vi "16bitImageglobal.vi"(4 "Enum":T3(ring), 5 "Palette Number (gray)":T1(ring), 7 "plane":u32, 8 "router":u8) -> (0 "Palette Number (gray) 2":T1(ring), 1 "Title":string, 2 "error out":errorcluster, 3 "Image Out (duplicate)":T2)   [LabVIEW 2009]
uses:
  <vilib>/vision/Image Controls.llb/IMAQ Image.ctl
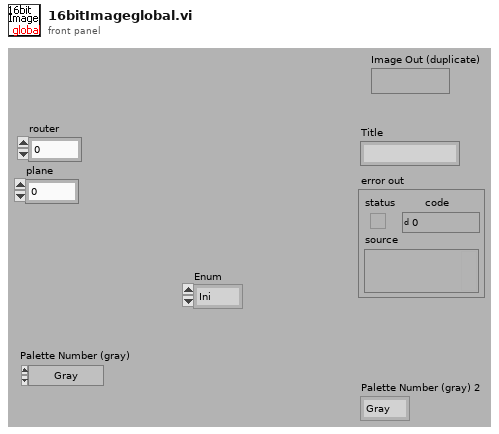
[diagram p1: front panel]
types:
  T1 = enum32{"Gray", "Binary", "Gradient", "Rainbow", "Temperature"}
  T2 = typedef "IMAQ Image.ctl" = refnum<image>
  T3 = enum16{"Ini", "Dump", "Colorpal", "Input", "Get"}
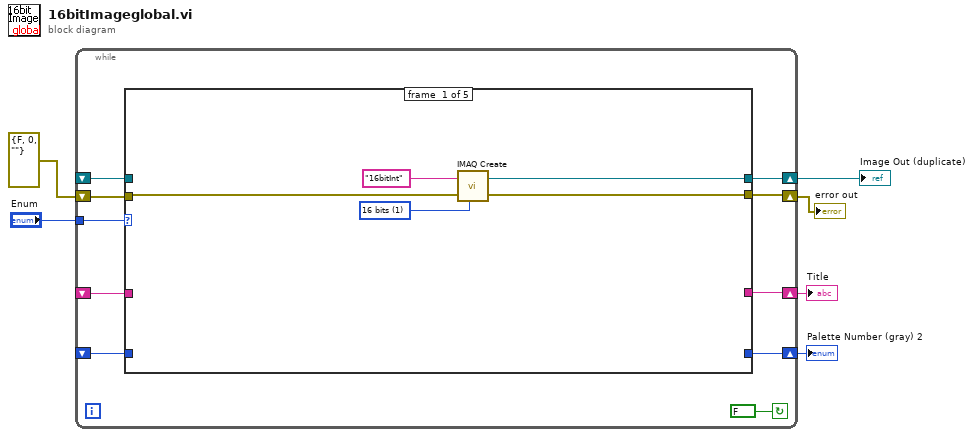
[diagram p0: block diagram]
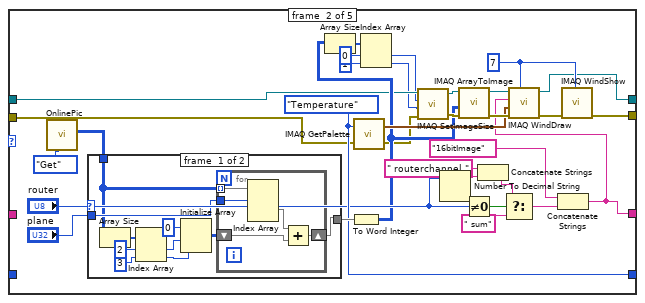
[diagram p2: hidden frame]
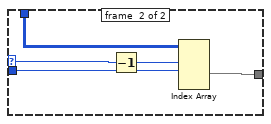
[diagram p3: hidden frame]
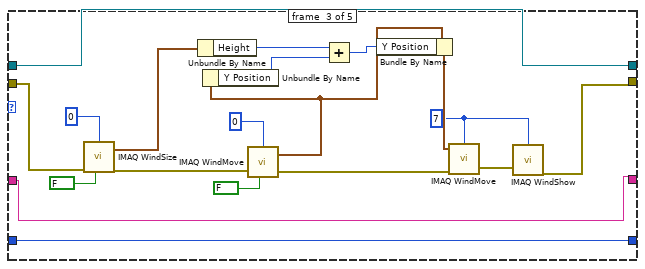
[diagram p4: hidden frame]
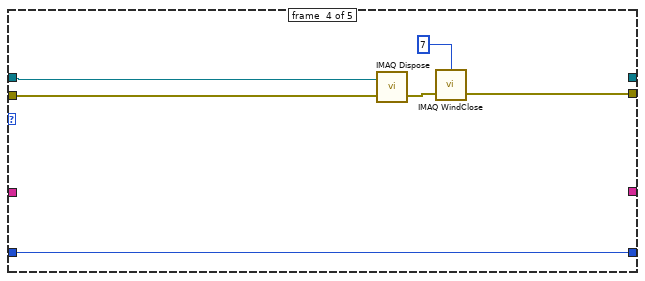
[diagram p5: hidden frame]
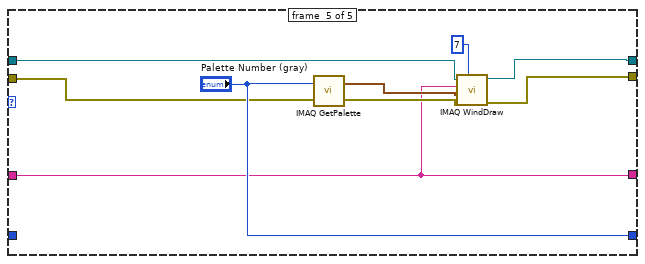
[diagram p6: hidden frame]
diagram:
  n1 = while {
    shift-right: [w13] -> w1
    shift-left: _ -> [w14]
    tunnel: "Enum" -> [w15]
    shift-right: [w12] -> w5
    shift-left: _ -> [w11]
    shift-right: [w10] -> w4
    shift-left: _ -> [w9]
    shift-right: [w8] -> w3
    shift-left: errorcluster {"status"=FALSE, "code"=0, "source"=""} ("error out") -> [w7]
    stop <- FALSE continue-if-true
    n2 = case shown="\"Input\"" w15 {
      tunnel: w14 -> [_ w26 w80 w96 w107]
      tunnel: [w19 w45 w80 _ w104] -> w13
      tunnel: [w18 w48 w78 w98 w105] -> w8
      tunnel: [_ w33 w76 _ w100] -> w12
      tunnel: w11 -> [_ _ w76 _ w100]
      tunnel: [_ w42 w75 w94 "Palette Number (gray)"] -> w10
      tunnel: w9 -> [_ _ w75 w94 _]
      tunnel: w7 -> [w17 w32 w74 w93 w99]
      frame #0 {
        w20 = u32 1 items=["8 bits", "16 bits", "Float", "Complex", "RGB", "HSL"] ("Image Type")
        n3 = call "IMAQ Create"("Image Name"="16bitInt", "Image Type"=w20, "error in (no error)"=w17) -> ("New Image"=w19:T2, "error out"=w18:errorcluster)  [unwired: 2 in]
      }
      frame #1 {
        w42 = T1."Temperature" ("Palette Number (gray)")
        w46 = 7 ("Window Number (0...15)")
        n4 = call "OnlinePic.vi"("action"=enum16{"Get", "Set", "Change", "ini"}."Get" ("Enum")) -> ("Sum of Photons"=w49:u32[][][][])  [unwired: 6 in, 4 out]
        n5 = case shown="0" "router" {
          selector: "router" -> [_ w70]
          tunnel: "plane" -> [w63 w73]
          tunnel: w49 -> [w54 w72]
          tunnel: [w62 w71] -> w44
          frame #0 {
            n6 = Array Size(array=w54) -> (size(s)=w57:i32[])
            n7 = Index Array(array=w57, index #1=2 ("index"), index #2=3 ("index")) -> (element #1=w56:i32, element #2=w55:i32)
            n8 = Initialize Array(u32 0, w56, w55) -> (w61:u32[][])
            n9 = for {
              tunnel: w54 -> [w68] mode=indexing
              shift-right: [w64] -> w62
              shift-left: w61 -> [w65]
              tunnel: w63 -> [w67]
              n10 = Index Array(array=w68, index (dim 0)=w67) -> (element=w66:u32[][])  [unwired: 2 in]
              n11 = Add(x=w66, y=w65) -> (x+y=w64:u32[][])
            }
          }
          frame #1 {
            n12 = Decrement(x=w70) -> (x-1=w69:u8)
            n13 = Index Array(array=w72, index (dim 0)=w69, index (dim 1)=w73) -> (element=w71:u32[][])  [unwired: 2 in]
          }
        }
        n14 = To Word Integer(number=w44) -> (16bit integer=w28:i16[][])
        n15 = Array Size(array=w28) -> (size(s)=w29:i32[])
        n16 = call "IMAQ GetPalette"("Palette Number (gray)"=w42, "error in (no error)"=w32) -> ("Color Palette"=w43:cluster{"Red":u8, "Green":u8, "Blue":u8}[], "error out"=w27:errorcluster)  [unwired: 3 in]
        n17 = Index Array(array=w29, index #1=0 ("index"), index #2=1 ("index")) -> (element #1=w23:i32, element #2=w22:i32)
        n18 = call "IMAQ SetImageSize"("error in (no error)"=w27, "Y Resolution"=w22, "X Resolution"=w23, "Image"=w26) -> ("error out"=w31:errorcluster, "Image Out"=w30:T2)  [unwired: 1 in]
        n19 = Number To Decimal String(number="router") -> (decimal integer string=w38:string)  [unwired: 1 in]
        n20 = call "IMAQ ArrayToImage"("error in (no error)"=w31, "Image Pixels (I16)"=w28, "Image"=w30) -> ("error out"=w51:errorcluster, "Image Out"=w50:T2)  [unwired: 7 in]
        n21 = Not Equal To 0?(x="router") -> (x != 0?=w41:bool)
        n22 = Concatenate Strings(" routerchannel " ("string"), w38) -> (w39:string)
        n23 = Select(t=w39, s=w41, f=" sum") -> (s? t:f=w35:string)
        n24 = Concatenate Strings("16bitImage" ("Title"), w35) -> (w33:string)
        n25 = call "IMAQ WindDraw"("Window Number (0...15)"=w46, "error in (no error)"=w51, "Color Palette"=w43, "Title"=w33, "Image"=w50) -> ("error out"=w47:errorcluster, "Image Out (duplicate)"=w45:T2)  [unwired: 5 in]
        n26 = call "IMAQ WindShow"("error in (no error)"=w47, "Window Number (0...15)"=w46) -> ("error out"=w48:errorcluster)  [unwired: 4 in, 2 out]
      }
      frame #2 {
        w77 = 7 ("Window Number (0...15)")
        n27 = call "IMAQ WindSize"("error in (no error)"=w74, "Get/Set Status? (Set)"=FALSE, "Window Number"=0) -> ("error out"=w87:errorcluster, "Width & Height out"=w85:cluster{"Width":i32, "Height":i32})  [unwired: 3 in, 1 out]
        n28 = Unbundle By Name(w85) -> ("Height"=w84:i32)
        n29 = call "IMAQ WindMove"("Window Number (0...15)"=0, "Get/Set Status? (Set)"=FALSE, "error in (no error)"=w87) -> ("Coordinates (screen)"=w81:cluster{"X Position":i32, "Y Position":i32}, "error out"=w88:errorcluster)  [unwired: 2 in]
        n30 = Unbundle By Name(w81) -> ("Y Position"=w83:i32)
        n31 = Add(x=w84, y=w83) -> (x+y=w82:i32)
        n32 = Bundle By Name(cluster=w81, "Y Position"=w82) -> (w86:cluster{"X Position":i32, "Y Position":i32})
        n33 = call "IMAQ WindMove"("Window Number (0...15)"=w77, "Coordinates (screen)"=w86, "error in (no error)"=w88) -> ("error out"=w79:errorcluster)  [unwired: 2 in, 1 out]
        n34 = call "IMAQ WindShow"("error in (no error)"=w79, "Window Number (0...15)"=w77) -> ("error out"=w78:errorcluster)  [unwired: 4 in, 2 out]
      }
      frame #3 {
        n35 = call "IMAQ Dispose"("Image"=w96, "error in (no error)"=w93) -> ("error out"=w97:errorcluster)  [unwired: 4 in]
        n36 = call "IMAQ WindClose"("Window Number (0...15)"=7, "error in (no error)"=w97) -> ("error out"=w98:errorcluster)  [unwired: 4 in]
      }
      frame #4 {
        n37 = call "IMAQ GetPalette"("Palette Number (gray)"="Palette Number (gray)", "error in (no error)"=w99) -> ("Color Palette"=w102:cluster{"Red":u8, "Green":u8, "Blue":u8}[], "error out"=w101:errorcluster)  [unwired: 3 in]
        n38 = call "IMAQ WindDraw"("Window Number (0...15)"=7, "error in (no error)"=w101, "Color Palette"=w102, "Title"=w100, "Image"=w107) -> ("error out"=w105:errorcluster, "Image Out (duplicate)"=w104:T2)  [unwired: 5 in]
      }
    }
  }
  "error out" <- w3
  "Title" <- w5
  "Image Out (duplicate)" <- w1
  "Palette Number (gray) 2" <- w4
